vi "Image_Create_1D_Bayer_Array.vi"(8 "error in (no error)":errorcluster, 10 "Image Configuration":T1={"Width"=1920, "Height"=1080}, 11 "Bayer Pattern":u16[][](array[numeric])=[[1, 2], [0, 1]]) -> (0 "error out":errorcluster, 3 "Bayer Pattern 1D Array":u16[](array[numeric]))   [LabVIEW 2020]
uses:
  ctl/Image_Configuration.ctl
panel:
  # "R:0\nG:1\nB:2\nC:3"
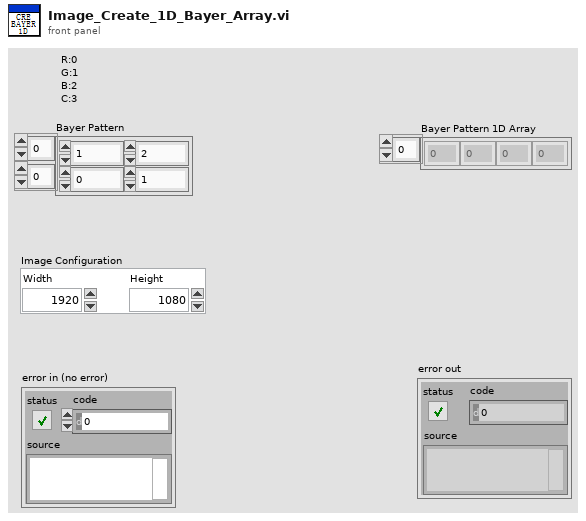
[diagram p1: front panel]
types:
  T1 = typedef "Image_Configuration.ctl" = cluster{"Width":i32, "Height":i32}
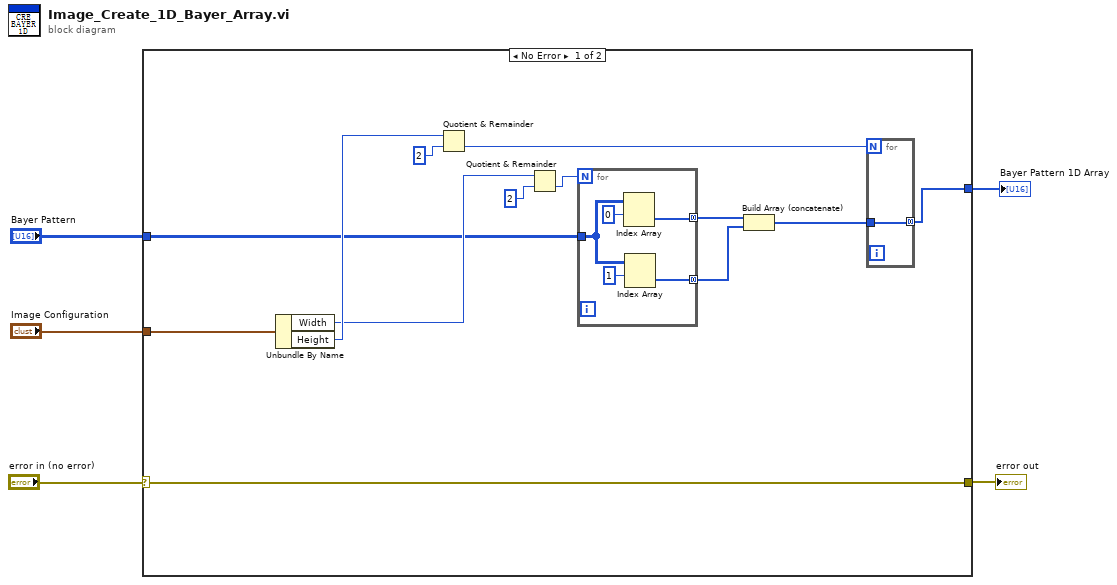
[diagram p0: block diagram]
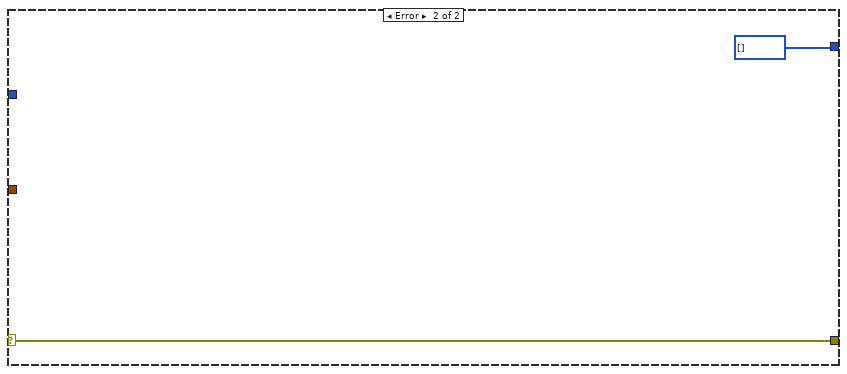
[diagram p2: hidden frame]
diagram:
  n1 = case shown="No Error" "error in (no error)" {
    selector: "error in (no error)" -> [w18 w26]
    tunnel: "Image Configuration" -> [w8 _]
    tunnel: "Bayer Pattern" -> [w7 _]
    tunnel: [w18 w26] -> w2
    tunnel: [w6 u16[] []] -> w1
    frame No Error {
      n2 = Unbundle By Name(w8) -> ("Width"=w15:i32, "Height"=w17:i32)
      n3 = Quotient & Remainder(x=w17, y=2) -> (floor(x/y)=w14:i32)  [unwired: 1 out]
      n4 = Quotient & Remainder(x=w15, y=2) -> (floor(x/y)=w16:i32)  [unwired: 1 out]
      n5 = for {
        N: w16 -> [_]
        tunnel: w7 -> [w24]
        tunnel: [w21] -> w13 mode=concatenating
        tunnel: [w20] -> w12 mode=concatenating
        n6 = Index Array(array=w24, index (row)=0) -> (element=w21:u16[])  [unwired: 1 in]
        n7 = Index Array(array=w24, index (row)=1) -> (element=w20:u16[])  [unwired: 1 in]
      }
      n8 = Build Array (concatenate)(w13, w12) -> (w11:u16[])
      n9 = for {
        N: w14 -> [_]
        tunnel: w11 -> [w19]
        tunnel: [w19] -> w6 mode=concatenating
      }
    }
    frame Error {
    }
  }
  "error out" <- w2
  "Bayer Pattern 1D Array" <- w1
